vi "Remove Key.vi"(7 "Section Name":string, 8 "error in (no error)":errorcluster, 10 "Key Name":string, 11 "Config in":T1) -> (0 "error out":errorcluster, 2 "Key Found?":bool, 3 "Config out":T1)   [LabVIEW 2022 SP3, in "LabVIEW-Config.lvlib"]
uses:
  LabVIEW-Config.lvlib
  Config.ctl
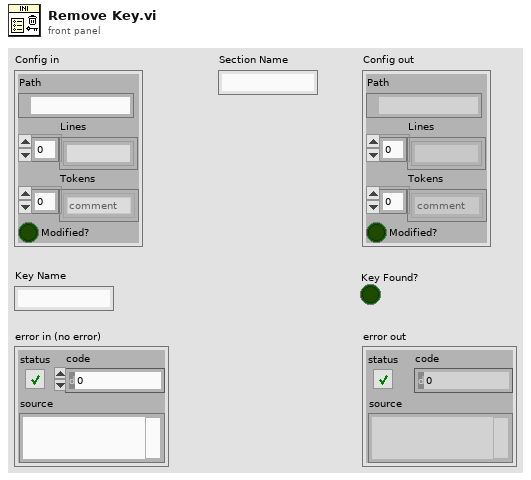
[diagram p1: front panel]
types:
  T1 = typedef "LabVIEW-Config.lvlib/Config.ctl" = cluster{"Path":path, "Lines":string[], "Tokens":enum8{"comment", "section", "key"}[], "Modified?":bool}
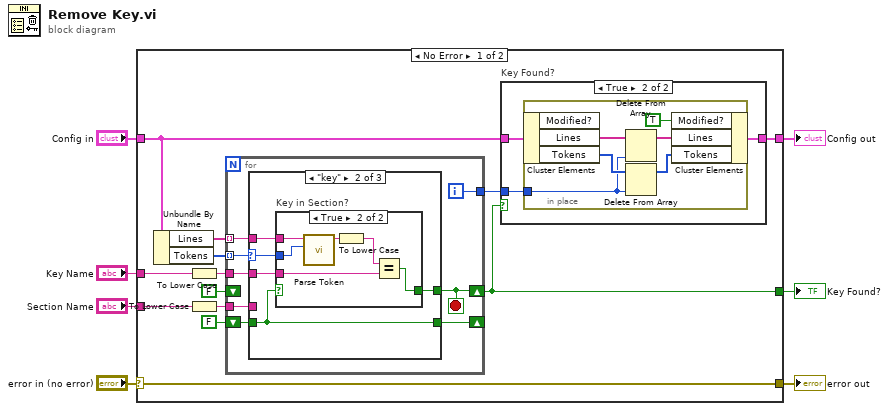
[diagram p0: block diagram]
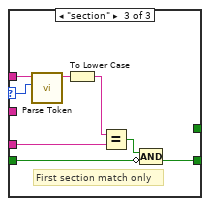
[diagram p4: hidden frame]
diagram:
  n1 = case shown="No Error" "error in (no error)" {
    selector: "error in (no error)" -> [w18 w60]
    tunnel: "Config in" -> [w12 w59]
    tunnel: [w18 w60] -> w6
    tunnel: [w13 w59] -> w4
    tunnel: "Section Name" -> [w17 _]
    tunnel: [w9 _] -> w2
    tunnel: "Key Name" -> [w11 _]
    frame No Error {
      n2 = Unbundle By Name(w12) -> ("Lines"=w19:string[], "Tokens"=w20:enum8{"comment", "section", "key"}[])
      n3 = To Lower Case(string=w11) -> (all lower case string=w10:string)
      n4 = To Lower Case(string=w17) -> (all lower case string=w16:string)
      n5 = for {
        tunnel: w20 -> [w28] mode=indexing
        tunnel: w19 -> [w27] mode=indexing
        tunnel: w16 -> [w26]
        shift-right: [w24] -> _
        shift-left: FALSE -> [w25]
        shift-right: [w22] -> w9
        shift-left: FALSE -> [_]
        tunnel: w10 -> [w23]
        tunnel: [w21] -> w8
        i -> [w21]
        stop <- w22 stop-if-true
        n6 = case shown="\"key\"" w28 {
          selector: w28 -> [_ w30 w42]
          tunnel: w27 -> [_ w34 w43]
          tunnel: w26 -> [_ _ w48]
          tunnel: [w29 w33 w44] -> w24
          tunnel: w25 -> [w29 w33 w46]
          tunnel: w23 -> [_ w32 _]
          tunnel: [_ w31 _] -> w22
          frame "comment" {
          }
          frame "key" {
            n7 = case "Key in Section?" shown="True" w33 {
              tunnel: w34 -> [_ w37]
              tunnel: w32 -> [_ w40]
              tunnel: [_ w38] -> w31
              tunnel: w30 -> [_ w36]
              frame False {
              }
              frame True {
                n8 = call "Parse Token.vi"("Token"=w36, "Line"=w37) -> ("Name"=w35:string)  [unwired: 8 in, 1 out]
                n9 = To Lower Case(string=w35) -> (all lower case string=w39:string)
                n10 = Equal?(x=w39, y=w40) -> (x = y?=w38:bool)
              }
            }
          }
          frame "section" {
            # "First section match only"
            n11 = call "Parse Token.vi"("Token"=w42, "Line"=w43) -> ("Name"=w41:string)  [unwired: 8 in, 1 out]
            n12 = To Lower Case(string=w41) -> (all lower case string=w47:string)
            n13 = Equal?(x=w47, y=w48) -> (x = y?=w45:bool)
            n14 = Compound Arithmetic op=AND(w45, invert w46) -> (w44:bool)
          }
        }
      }
      n15 = case "Key Found?" shown="True" w9 {
        tunnel: [w49 w52] -> w13
        tunnel: w12 -> [w49 w51]
        tunnel: w8 -> [_ w50]
        frame False {
        }
        frame True {
          n16 = in-place {
            in-place-border: w50 -> [w53]
            n17 = in-place-cluster #1(w51) -> ("Lines"=w57:string[], "Tokens"=w56:enum8{"comment", "section", "key"}[])  [unwired: 1 out]
            n18 = Delete From Array(array=w57, index=w53) -> (array with subset deleted=w54:string[])  [unwired: 1 in, 1 out]
            n19 = Delete From Array(array=w56, index=w53) -> (array with subset deleted=w55:enum8{"comment", "section", "key"}[])  [unwired: 1 in, 1 out]
            n20 = in-place-cluster #1("Modified?"=TRUE, "Lines"=w54, "Tokens"=w55) -> (w52:T1)
          }
        }
      }
    }
    frame Error {
    }
  }
  "error out" <- w6
  "Config out" <- w4
  "Key Found?" <- w2
